vi "Get Status Code.vi"(8 "error in (no error)":errorcluster, 11 "Response in":refnum<class "Response.lvclass">) -> (0 "error out":errorcluster, 2 "Status Code":u16, 3 "Response out":refnum<class "Response.lvclass">)   [LabVIEW 2020, in "HTTP Utils.lvlib" / "Response.lvclass"]
uses:
  Response.lvclass
  Response.lvclass/Response.ctl
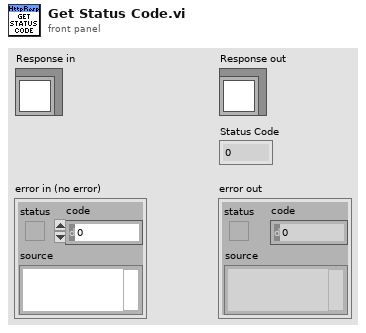
[diagram p1: front panel]
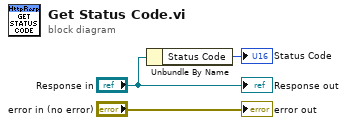
[diagram p0: block diagram]
diagram:
  n1 = Unbundle By Name("Response in") -> ("Status Code"=→"Status Code":u16)
  "error out" <- "error in (no error)"
  "Response out" <- "Response in"
